vi "Clear Specific Error.vi"(7 "code":i32, 8 "error in (no error)":errorcluster) -> (0 "error out":errorcluster)   [LabVIEW 2011]
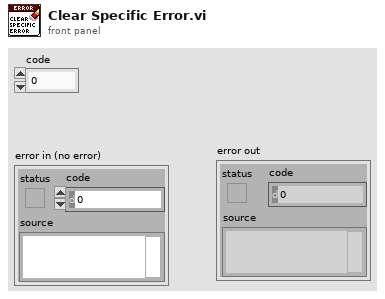
[diagram p1: front panel]
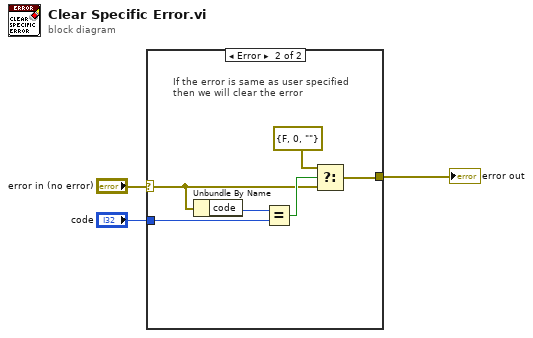
[diagram p0: block diagram]
diagram:
  n1 = case shown="Error" "error in (no error)" {
    selector: "error in (no error)" -> [w4 w7]
    tunnel: [w4 w6] -> w2
    tunnel: "code" -> [_ w9]
    frame No Error {
    }
    frame Error {
      # "If the error is same as user specified\nthen we will clear the error"
      n2 = Unbundle By Name(w7) -> ("code"=w10:i32)
      n3 = Equal?(x=w10, y=w9) -> (x = y?=w8:bool)
      n4 = Select(t=errorcluster {"status"=FALSE, "code"=0, "source"=""}, s=w8, f=w7) -> (s? t:f=w6:errorcluster)
    }
  }
  "error out" <- w2
